vi "SaveCurrentState.vi"(8 "error in (no error)":errorcluster, 10 "Current State":string, 11 "Byte Stream File in":refnum<file>) -> (0 "error out":errorcluster)   [LabVIEW 2020]
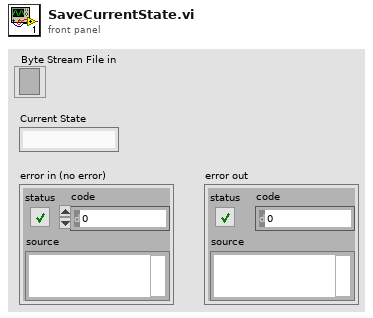
[diagram p1: front panel]
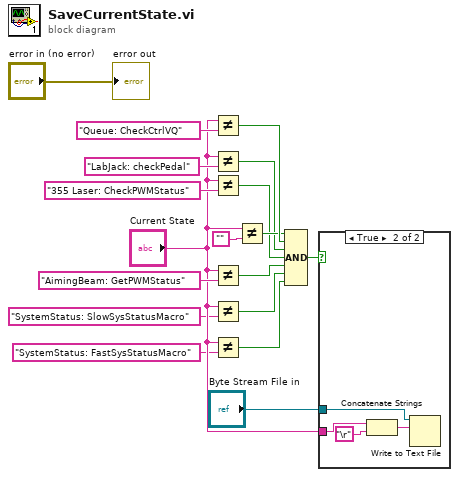
[diagram p0: block diagram]
diagram:
  n1 = Not Equal?(x="Current State", y="Queue: CheckCtrlVQ" ("State(s) in Front (\"\")")) -> (x != y?=w15:bool)
  n2 = Not Equal?(x="Current State", y="LabJack: checkPedal") -> (x != y?=w10:bool)
  n3 = Not Equal?(x="Current State", y="355 Laser: CheckPWMStatus") -> (x != y?=w9:bool)
  n4 = Not Equal?(x="Current State", y="AimingBeam: GetPWMStatus") -> (x != y?=w7:bool)
  n5 = Not Equal?(x="Current State", y="SystemStatus: SlowSysStatusMacro") -> (x != y?=w3:bool)
  n6 = Not Equal?(x="Current State", y="SystemStatus: FastSysStatusMacro") -> (x != y?=w2:bool)
  n7 = Not Equal?(x="Current State", y="" ("Empty String Constant")) -> (x != y?=w14:bool)
  n8 = Compound Arithmetic op=AND(w14, w15, w10, w9, w7, w3, w2) -> (w12:bool)
  n9 = case shown="True" w12 {
    tunnel: "Byte Stream File in" -> [_ w22]
    tunnel: "Current State" -> [_ w19]
    frame False {
    }
    frame True {
      n10 = Concatenate Strings(w19, "\r" ("Carriage Return Constant")) -> (w20:string)
      n11 = Write to Text File(file (use dialog)=w22, text=w20) -> ()  [unwired: 2 in, 3 out]
    }
  }
  "error out" <- "error in (no error)"
